vi "Get Public API.vi"(8 "error in (no error)":errorcluster, 11 "Instrument.Example In":refnum<class "Instrument.Example.lvclass">) -> (0 "error out":errorcluster, 2 "Commands":string[](array[string]), 3 "Instrument.Example out":refnum<class "Instrument.Example.lvclass">)   [LabVIEW 2016, in "Instrument.Example.lvclass"]
uses:
  Instrument.Example.lvclass
  <userlib>/LevyLab/Levylab Instruments/SMOs/Instrument/Instrument.lvclass
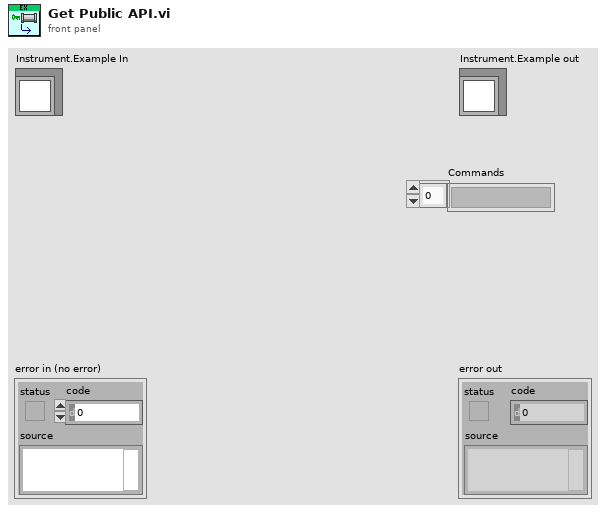
[diagram p1: front panel]
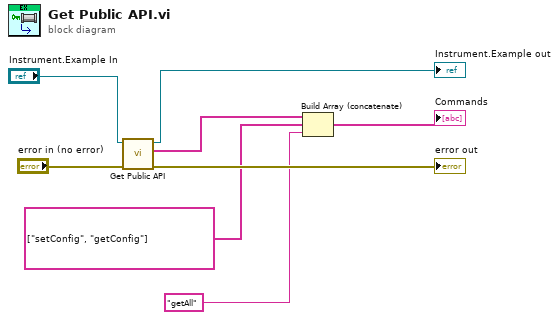
[diagram p0: block diagram]
diagram:
  n1 = call-parent "Get Public API.vi"("error in (no error)"="error in (no error)", "Instrument in"="Instrument.Example In") -> ("error out"=→"error out":errorcluster, "Commands"=w4:string[], "Instrument out"=→"Instrument.Example out":refnum<class "Instrument.Example.lvclass">)  [unwired: 7 in]
  n2 = Build Array (concatenate)(w4, string[] ["setConfig", "getConfig"] ("element"), "getAll" ("Command")) -> (→"Commands":string[])
